vi "Enable disable control.vi"(10 "Enabled?":bool, 11 "Digital in":refnum<vi>) -> ()   [LabVIEW 2019, in "Panther Dashboard.lvlib"]
uses:
  Panther Dashboard.lvlib
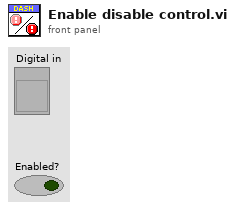
[diagram p1: front panel]
types:
  T1 = enum8{"Enabled", "Disabled", "Disabled and Grayed Out"}
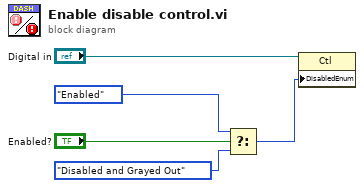
[diagram p0: block diagram]
diagram:
  n1 = Select(t=T1."Enabled" ("Disabled"), s="Enabled?", f=T1."Disabled and Grayed Out") -> (s? t:f=w5:T1)
  n2 = property on="Property Node" class="Ctl"(reference="Digital in", "DisabledEnum"=w5) -> ()  [unwired: 1 in, 2 out]
